vi "sub_value changed.vi"(0 "输入":dbl) -> (3 "值改变":bool, 4 "值不变":bool)   [LabVIEW 2015]
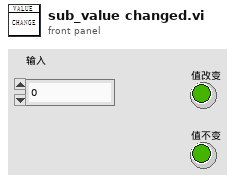
[diagram p1: front panel]
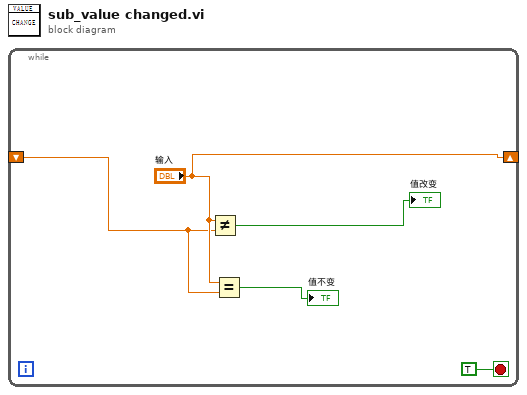
[diagram p0: block diagram]
diagram:
  n1 = while {
    shift-right: ["输入"] -> _
    shift-left: _ -> [w2]
    stop <- TRUE stop-if-true
    n2 = Not Equal?(x="输入", y=w2) -> (x != y?=→"值改变":bool)
    n3 = Equal?(x="输入", y=w2) -> (x = y?=→"值不变":bool)
  }
